vi "求角度.vi"(7 "Line form":enum16{"Line", "Two Point"}(ring)=enum."Two Point", 9 "Point 2":cluster{"X":sgl, "Y":sgl}, 10 "Point 1":cluster{"X":sgl, "Y":sgl}, 11 "Line":T1) -> (3 "Line Data":cluster{"X":sgl, "Y":sgl, "T":sgl})   [LabVIEW 2015]
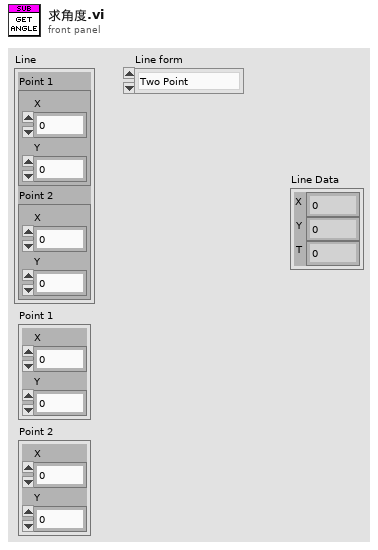
[diagram p1: front panel]
types:
  T1 = cluster{"Point 1":cluster{"X":sgl, "Y":sgl}, "Point 2":cluster{"X":sgl, "Y":sgl}}
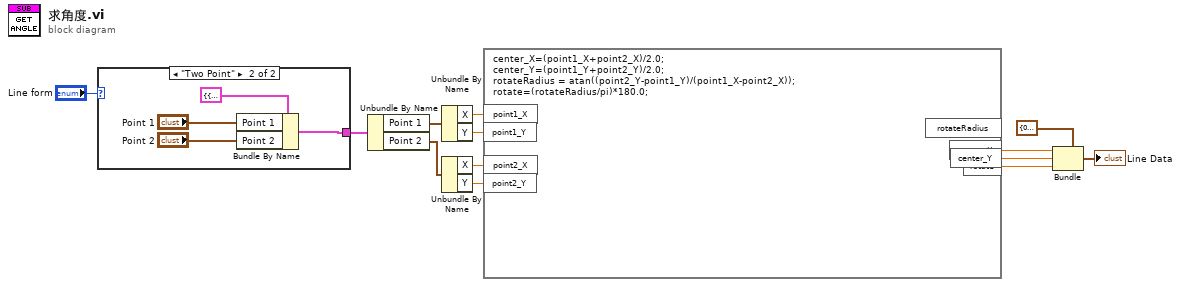
[diagram p0: block diagram]
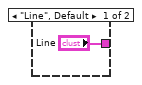
[diagram p2: hidden frame]
diagram:
  n1 = case shown="\"Two Point\"" "Line form" {
    tunnel: ["Line" w15] -> w10
    frame "Line", Default {
    }
    frame "Two Point" {
      n2 = Bundle By Name(cluster=T1 {"Point 1"={"X"=0.0, "Y"=0.0}, "Point 2"={"X"=0.0, "Y"=0.0}} ("Line"), "Point 1"="Point 1", "Point 2"="Point 2") -> (w15:T1)
    }
  }
  n3 = Unbundle By Name(w10) -> ("Point 1"=w12:cluster{"X":sgl, "Y":sgl}, "Point 2"=w13:cluster{"X":sgl, "Y":sgl})
  n4 = Unbundle By Name(w12) -> ("X"=w8:sgl, "Y"=w7:sgl)
  n5 = Unbundle By Name(w13) -> ("X"=w6:sgl, "Y"=w5:sgl)
  n6 = formula code="center_X=(point1_X+point2_X)/2.0;\ncenter_Y=(point1_Y+point2_Y)/2.0;\nrotateRadius = atan((point2_Y-point1_Y)/(point1_X-point2_X));\nrotate=(rotateRadius/pi)*180.0;"("point1_X"=w8, "point1_Y"=w7, "point2_X"=w6, "point2_Y"=w5) -> ("rotate"=w2:dbl, "center_X"=w4:dbl, "center_Y"=w3:dbl)  [unwired: 1 out]
  n7 = Bundle(cluster=cluster{"X":sgl, "Y":sgl, "T":sgl} {"X"=0.0, "Y"=0.0, "T"=0.0} ("Line Data 2"), "X"=w4, "Y"=w3, "T"=w2) -> (→"Line Data":cluster{"X":sgl, "Y":sgl, "T":sgl})
